vi "Actor Core.vi"(8 "error in":errorcluster, 11 "ListboxBusMonitorPanel in":refnum<class "ListboxBusMonitorPanel.lvclass">) -> (0 "error out":errorcluster, 3 "Actor out":refnum<class "Actor.lvclass">)   [LabVIEW 2020, in "ListboxBusMonitor.lvlib" / "ListboxBusMonitorPanel.lvclass"]
doc: "(<B>Filename</B>: Actor Framework.lvlib:Actor.lvclass:Actor Core.vi)\n\nReceives messages to the actor, reacts to them, and initiates any error handling that may shut the actor down.\n\nDescendant classes may override this VI to append parallel tasks for the actor to complete while it handles messages. Overrides use the Call Parent Method node."
uses:
  <vilib>/gpm_packages/@cs/BusMonitor/ListboxBusMonitor/ListboxBusMonitorPanel/ListboxBusMonitorPanel.lvclass
  <vilib>/ActorFramework/Actor/Actor.lvclass
  <vilib>/gpm_packages/@cs/BusMonitor/ListboxBusMonitor/ListboxBusMonitorPanel/ListboxBusMonitorPanel.lvclass/ListboxBusMonitorPanel.ctl
  <vilib>/gpm_packages/@cs/listbox/ListboxExtensions.lvlib
panel:
  in  "Multicolumn Listbox":i32(listbox)
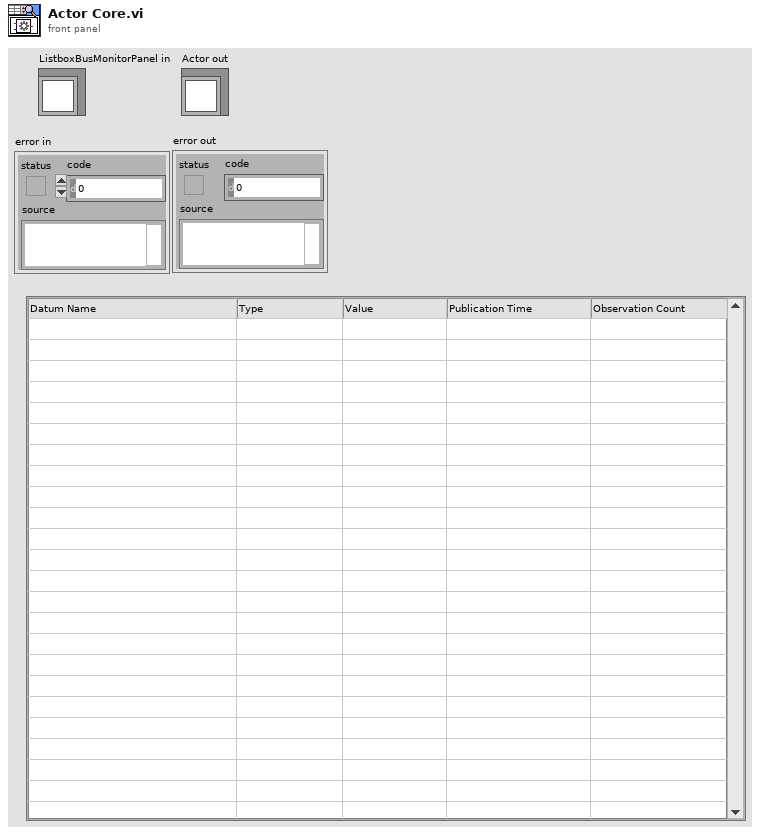
[diagram p1: front panel]
types:
  T1 = enum32{"Invalid", "Standard", "Closed", "Hidden", "Minimized", "Maximized"}
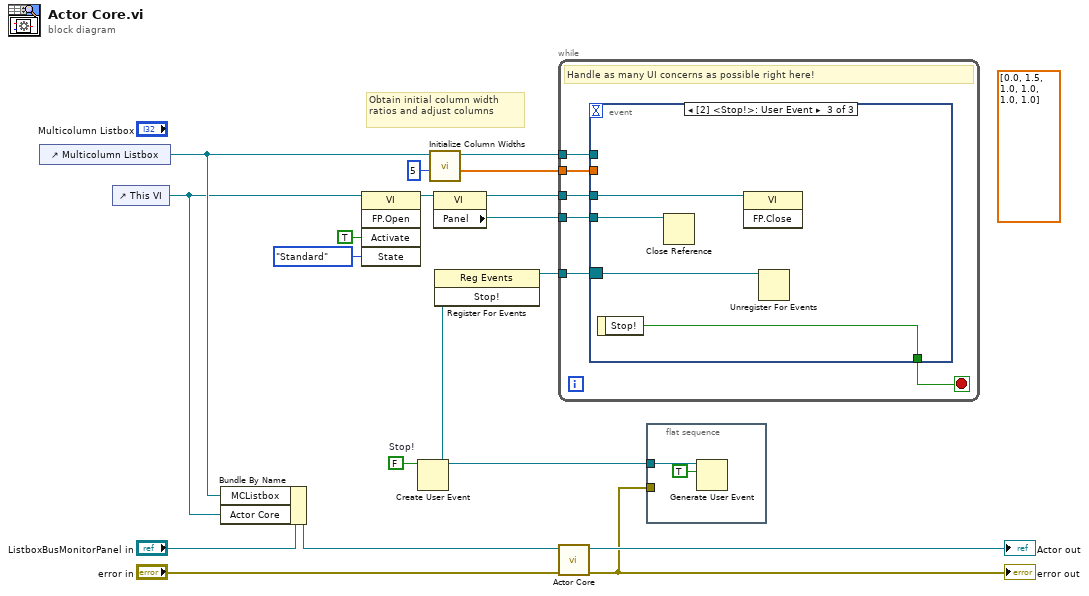
[diagram p0: block diagram]
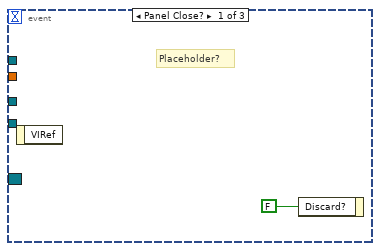
[diagram p2: hidden frame]
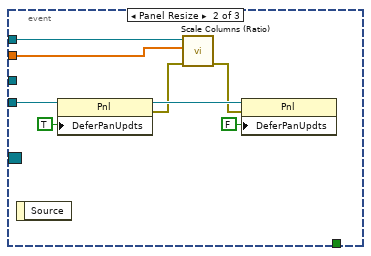
[diagram p3: hidden frame]
diagram:
  (unwired) dbl[] [0.0, 1.5, 1.0, 1.0, 1.0, 1.0] ("Column Widths (Ratio)")
  w14 = FALSE  # Stop!
  # "Obtain initial column width\nratios and adjust columns"
  n1 = control-ref of="Multicolumn Listbox"() -> (w11:refnum<vi>)
  n2 = control-ref of="This VI"() -> (w8:refnum<vi>)
  n3 = Bundle By Name(cluster="ListboxBusMonitorPanel in", "MCListbox"=w11, "Actor Core"=w8) -> (w1:refnum<class "ListboxBusMonitorPanel.lvclass">)
  n4 = invoke class="VI" method="FP.Open"(reference=w8, "Activate"=TRUE ("Activate?"), "State"=T1."Standard") -> (reference out=w4:refnum<vi>)  [unwired: 2 in, 4 out]
  n5 = Create User Event(user event datatype=w14) -> (user event=w13:refnum<user-event>)  [unwired: 1 in, 1 out]
  n6 = call <vilib>:"Initialize Column Widths.vi"("Number of Columns"=5 ("Number of Columns (including header)"), "MCListbox Reference"=w11) -> ("Column Widths (Ratio)"=w5:dbl[], "MCListbox Reference Out"=w10:refnum<vi>)  [unwired: 8 in]
  n7 = property class="VI"(reference=w4) -> (reference out=w7:refnum<vi>, "Panel"=w6:refnum<vi>)  [unwired: 1 in, 1 out]
  n8 = register-events(w13) -> (reference out=w15:refnum<event-registration>)  [unwired: 2 in, 1 out]
  n9 = while {
    tunnel: w15 -> [w24]
    tunnel: w10 -> [w22]
    tunnel: w5 -> [w21]
    tunnel: w7 -> [w20]
    tunnel: w6 -> [w19]
    stop <- w23 stop-if-true
    # "Handle as many UI concerns as possible right here!"
    n10 = event shown="[2] <Stop!>: User Event" {
      selector: w24 -> [_ _ w36]
      dyn-events: _ -> [_ _ _]
      timeout: _ -> [_ _ _]
      tunnel: [_ _ w37] -> w23
      tunnel: w22 -> [_ w32 _]
      tunnel: w21 -> [_ w31 _]
      tunnel: w20 -> [_ _ w35]
      tunnel: w19 -> [_ w30 w34]
      event Panel Close? {
        # "Placeholder?"
        n11 = event-data() -> ()  [unwired: 1 in, 1 out]
        n12 = event-data("Discard?"=FALSE) -> ()  [unwired: 1 in, 1 out]
      }
      event Panel Resize {
        n13 = event-data() -> ()  [unwired: 1 in, 1 out]
        n14 = property class="Pnl"(reference=w30, "DeferPanUpdts"=TRUE ("Defer Panel Updates")) -> (reference out=w33:refnum<vi>, error out=w28:errorcluster)  [unwired: 1 in]
        n15 = call <vilib>:"Scale Columns (Ratio).vi"("error in (no error)"=w28, "Column Widths [unitless ratio]"=w31, "MulticolumnListbox in"=w32) -> ("error out"=w26:errorcluster)  [unwired: 8 in]
        n16 = property class="Pnl"(reference=w33, error in=w26, "DeferPanUpdts"=FALSE ("Defer Panel Updates")) -> ()  [unwired: 2 out]
      }
      event User Event {
        n17 = event-data() -> ("Stop!"=w37:bool)  [unwired: 1 in]
        n18 = Close Reference(reference=w34) -> ()  [unwired: 1 in, 1 out]
        n19 = invoke class="VI" method="FP.Close"(reference=w35) -> ()  [unwired: 2 in, 3 out]
        n20 = Unregister For Events(event registration refnum=w36) -> ()  [unwired: 1 in, 1 out]
      }
    }
  }
  n21 = call-parent "Actor Core.vi"("error in"="error in", "Actor in"=w1) -> ("error out"=w12:errorcluster, "Actor out"=→"Actor out":refnum<class "Actor.lvclass">)  [unwired: 8 in]
  "error out" <- w12
  n22 = flat-sequence {
    tunnel: w13 -> [w39]
    tunnel: w12 -> [_]
    frame #0 {
      n23 = Generate User Event(user event=w39, event data cluster=TRUE ("event data")) -> ()  [unwired: 2 in, 2 out]
    }
  }
